vi "Read.Construct.vi"(8 "error in (no error)":errorcluster, 9 "Refs":T1[](array[typedef]) format="%.0x", 10 "Parent":T1 format="%.0x", 11 "Read in":refnum<class "Read.lvclass">) -> (0 "error out":errorcluster, 3 "Read out":refnum<class "Read.lvclass">)   [LabVIEW 2015, in "Data Access API.lvlib" / "Read.lvclass"]
uses:
  Read.lvclass
  <vilib>/NI Veristand/Custom Device API/Custom Device Item Ref.ctl
  <vilib>/NI Veristand/Custom Device API/Data Access Type.ctl
  Read.lvclass/Read.ctl
  <vilib>/NI Veristand/Custom Device API/Custom Device API.lvlib
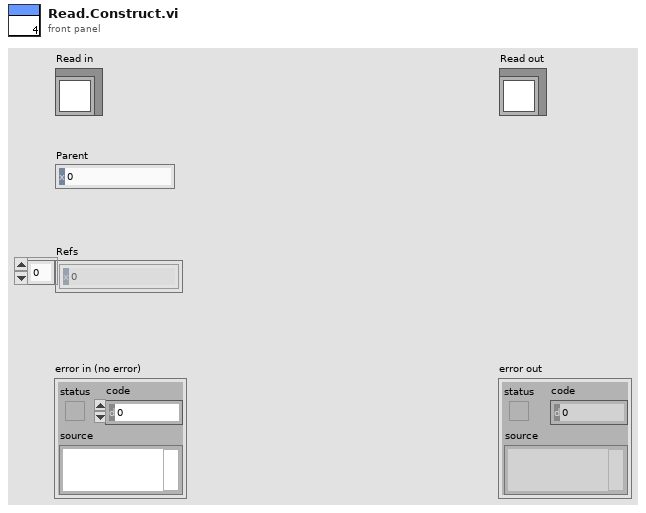
[diagram p1: front panel]
types:
  T1 = typedef "Custom Device API.lvlib/Custom Device Item Ref.ctl" = u64
  T2 = typedef "Custom Device API.lvlib/Data Access Type.ctl" = enum16{"Read", "Write"}
  T3 = typedef "Custom Device API.lvlib/Block Data Reference.ctl" = cluster{"Data Reference":T4, "Offset":u64, "Length":u64}
  T4 = typedef "Custom Device API.lvlib/Data Reference.ctl" = i32
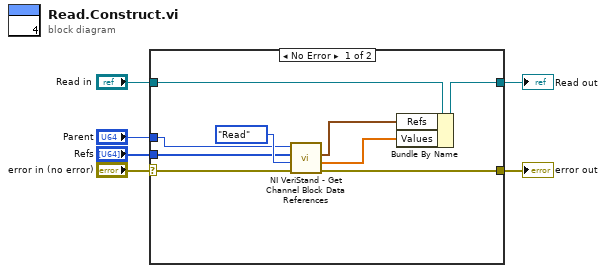
[diagram p0: block diagram]
diagram:
  n1 = case shown="No Error" "error in (no error)" {
    selector: "error in (no error)" -> [w12 w17]
    tunnel: [w11 w17] -> w5
    tunnel: [w14 w16] -> w3
    tunnel: "Read in" -> [w15 w16]
    tunnel: "Parent" -> [w8 _]
    tunnel: "Refs" -> [w7 _]
    frame No Error {
      n2 = call <vilib>:"NI VeriStand - Get Channel Block Data References.vi"("error in (no error)"=w12, "Access"=Data_Access_Type."Read", "Channel Refs"=w7, "Device Ref in"=w8) -> ("error out"=w11:errorcluster, "Values Array"=w9:dbl[], "Block Data Refs"=w10:T3[])  [unwired: 4 in, 1 out]
      n3 = Bundle By Name(cluster=w15, "Refs"=w10, "Values"=w9) -> (w14:refnum<class "Read.lvclass">)
    }
    frame Error {
    }
  }
  "error out" <- w5
  "Read out" <- w3
